vi "Before Run TS.vi"(8 "error in":errorcluster, 11 "DeepU Test Stand in":refnum<class "DeepU Test Stand.lvclass">) -> (0 "error out":errorcluster, 3 "DeepU Test Stand out":refnum<class "DeepU Test Stand.lvclass">)   [LabVIEW 2019, in "Test Stands.lvlib" / "DeepU Test Stand.lvclass"]
uses:
  DeepU Test Stand.lvclass
  C:/Users/wg/Documents/LV_Projects/test-stand/App/Generic Test Stand/Generic Test Stand.lvclass
  DAC/DeepU/Inverter/DAC Inverter.lvclass
  C:/Users/wg/Documents/LV_Projects/test-stand/App/DAC/DAC.lvclass
  Generic Test Stand/Generic Test Stand.lvclass/Generic Test Stand.ctl
  DeepU Test Stand.lvclass/DeepU Test Stand.ctl
  DAC/DAC.lvclass/DAC.ctl
  DAC/DAC.lvclass
  Generic Test Stand/Generic Test Stand.lvclass
  DAC/DeepU/FTCU/DAC FTCU.lvclass
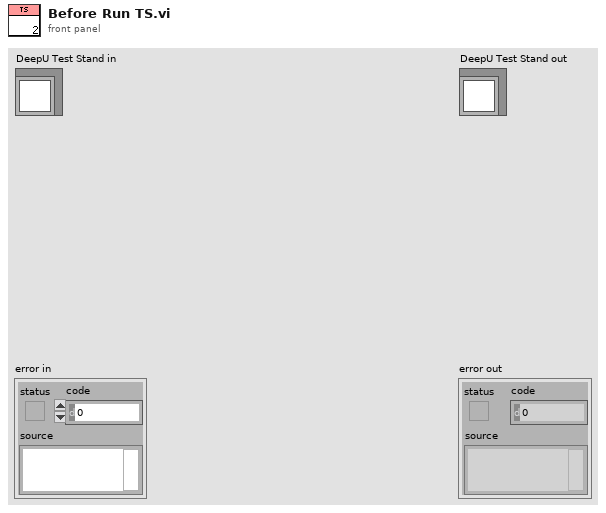
[diagram p1: front panel]
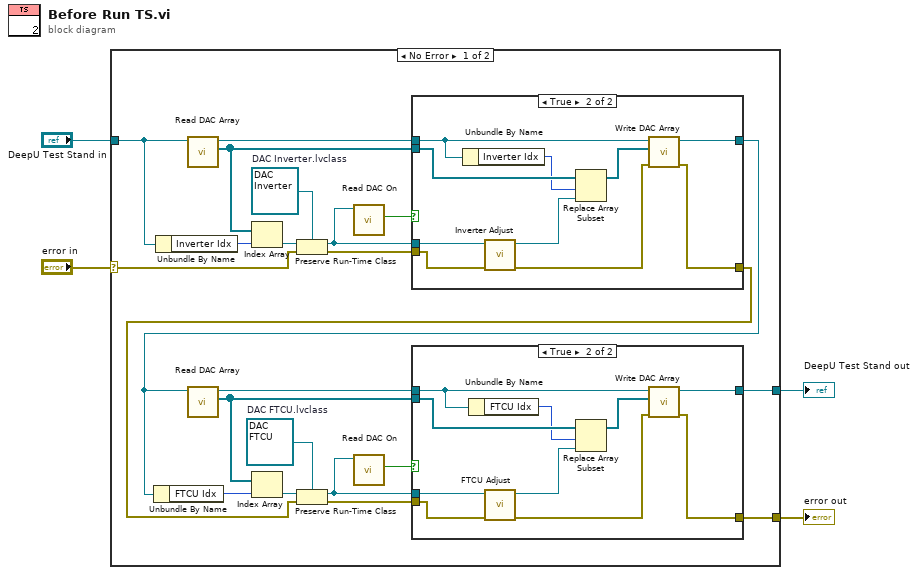
[diagram p0: block diagram]
diagram:
  n1 = case shown="No Error" "error in" {
    selector: "error in" -> [w12 w52]
    tunnel: [w6 w52] -> w1
    tunnel: [w7 w51] -> w2
    tunnel: "DeepU Test Stand in" -> [w13 w51]
    frame No Error {
      w5 = refnum<class "DAC FTCU.lvclass"> refnum  # DAC FTCU.lvclass
      w22 = refnum<class "DAC Inverter.lvclass"> refnum  # DAC Inverter.lvclass
      n2 = Unbundle By Name(w13) -> ("Inverter Idx"=w24:i32)
      n3 = call "Read DAC Array.vi"("Generic Test Stand in"=w13) -> ("DAC Array"=w19:refnum<class "DAC.lvclass">[], "Generic Test Stand out"=w25:refnum<class "DeepU Test Stand.lvclass">)  [unwired: 8 in, 1 out]
      n4 = Index Array(array=w19, index=w24) -> (element=w23:refnum<class "DAC.lvclass">)
      n5 = Preserve Run-Time Class(object in=w23, error in=w12, 2:w22) -> (object out=w21:refnum<class "DAC Inverter.lvclass">, error out=w20:errorcluster)
      n6 = call "Read DAC On.vi"("DAC in"=w21) -> ("DAC On"=w26:bool)  [unwired: 8 in, 2 out]
      n7 = case shown="True" w26 {
        tunnel: w25 -> [w40 w46]
        tunnel: [w40 w48] -> w10
        tunnel: w21 -> [_ w50]
        tunnel: w20 -> [w39 w49]
        tunnel: w19 -> [_ w47]
        tunnel: [w39 w41] -> w11
        frame False {
        }
        frame True {
          n8 = Unbundle By Name(w46) -> ("Inverter Idx"=w45:i32)
          n9 = call "Inverter Adjust.vi"("error in"=w49, "DAC Inverter in"=w50) -> ("error out"=w42:errorcluster, "DAC Inverter out"=w44:refnum<class "DAC Inverter.lvclass">)  [unwired: 8 in]
          n10 = Replace Array Subset(array=w47, new element=w44, index=w45) -> (w43:refnum<class "DAC.lvclass">[])
          n11 = call "Write DAC Array.vi"("error in (no error)"=w42, "DAC Array"=w43, "Generic Test Stand in"=w46) -> ("error out"=w41:errorcluster, "Generic Test Stand out"=w48:refnum<class "DeepU Test Stand.lvclass">)  [unwired: 7 in]
        }
      }
      n12 = Unbundle By Name(w10) -> ("FTCU Idx"=w15:i32)
      n13 = call "Read DAC Array.vi"("Generic Test Stand in"=w10) -> ("DAC Array"=w8:refnum<class "DAC.lvclass">[], "Generic Test Stand out"=w9:refnum<class "DeepU Test Stand.lvclass">)  [unwired: 8 in, 1 out]
      n14 = Index Array(array=w8, index=w15) -> (element=w16:refnum<class "DAC.lvclass">)
      n15 = Preserve Run-Time Class(object in=w16, error in=w11, 2:w5) -> (object out=w17:refnum<class "DAC FTCU.lvclass">, error out=w18:errorcluster)
      n16 = call "Read DAC On.vi"("DAC in"=w17) -> ("DAC On"=w14:bool)  [unwired: 8 in, 2 out]
      n17 = case shown="True" w14 {
        tunnel: w9 -> [w28 w34]
        tunnel: [w28 w36] -> w7
        tunnel: w17 -> [_ w38]
        tunnel: w18 -> [w27 w37]
        tunnel: w8 -> [_ w35]
        tunnel: [w27 w29] -> w6
        frame False {
        }
        frame True {
          n18 = Unbundle By Name(w34) -> ("FTCU Idx"=w33:i32)
          n19 = call "FTCU Adjust.vi"("error in"=w37, "DAC FTCU in"=w38) -> ("error out"=w30:errorcluster, "DAC FTCU out"=w32:refnum<class "DAC FTCU.lvclass">)  [unwired: 8 in]
          n20 = Replace Array Subset(array=w35, new element=w32, index=w33) -> (w31:refnum<class "DAC.lvclass">[])
          n21 = call "Write DAC Array.vi"("error in (no error)"=w30, "DAC Array"=w31, "Generic Test Stand in"=w34) -> ("error out"=w29:errorcluster, "Generic Test Stand out"=w36:refnum<class "DeepU Test Stand.lvclass">)  [unwired: 7 in]
        }
      }
    }
    frame Error {
    }
  }
  "error out" <- w1
  "DeepU Test Stand out" <- w2
